vi "Process Job.vi"(8 "error in (no error)":errorcluster, 10 "Task":refnum<class>, 11 "Cashier in":refnum<class "Cashier.lvclass">) -> (0 "error out":errorcluster, 3 "Cashier out":refnum<class "Cashier.lvclass">)   [LabVIEW 2023, in "Cashier.lvclass"]
doc: "Perform the task assigned by the work dispatcher. This VI is an override of a generic method all descendants of the Worker class must implement. \n\nThis method, being implemented by the Cashier class, handles the taking of an order from a Customer."
uses:
  Cashier.lvclass
  Order/Order.lvclass
  Customer Messages/Update order number Msg/Update order number Msg.lvclass/Update order number Msg.ctl
  <vilib>/ActorFramework/Message Enqueuer/Message Enqueuer.lvclass/Message Enqueuer.ctl
  Order/Order.lvclass/Order.ctl
  Customer Messages/Pick up Item Msg/Pick up Item Msg.lvclass
  c:/dev/_r/4/eng/lv-core/lvpostprocessingd/lv_mc_x86_64/dist_i386/vi.lib/ActorFramework/Message/Message.lvclass
  <vilib>/ActorFramework/Self-Addressed Msg/Self-Addressed Msg.lvclass/Self-Addressed Msg.ctl
  Work Dispatcher Messages/Add Task Msg/Add Task Msg.lvclass/Add Task Msg.ctl
  <vilib>/ActorFramework/Message Enqueuer/Enqueue.vi
  Customer Messages/Update order number Msg/Update order number Msg.lvclass
  Work Dispatcher Messages/Add Task Msg/Add Task Msg.lvclass
  <vilib>/ActorFramework/Message Priority Queue/Priority Enqueue.vi
  <vilib>/ActorFramework/Self-Addressed Msg/Self-Addressed Msg.lvclass
  Worker.lvclass
  Order/Order Item.lvclass
panel:
  in  "Ordered Item":string="Ordered item %d/%d..."
  in  "Taking Order":string="Taking order..."
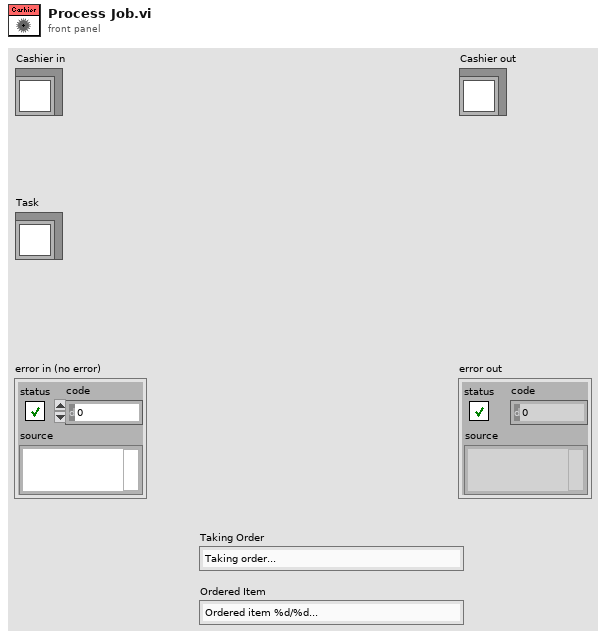
[diagram p1: front panel]
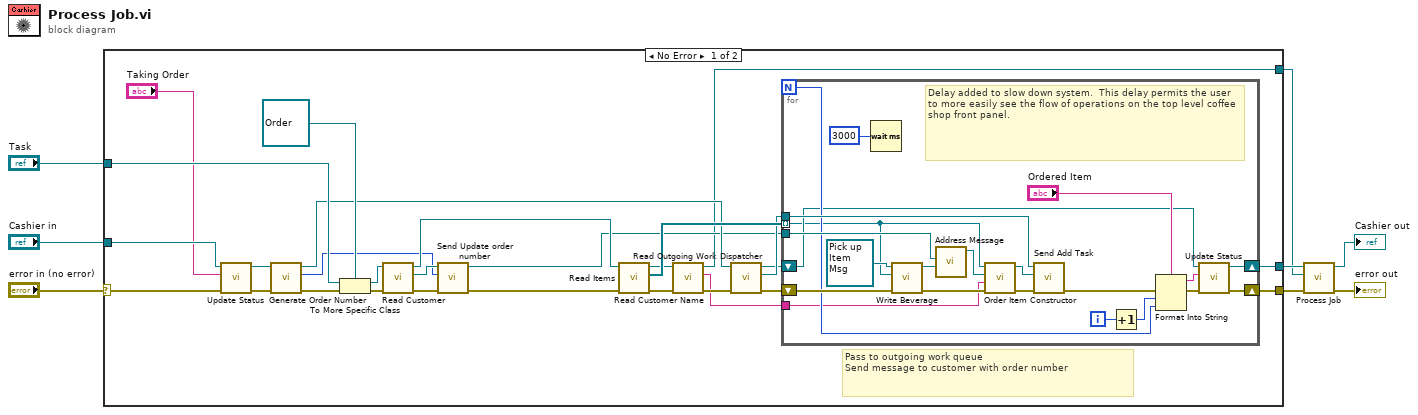
[diagram p0: block diagram]
diagram:
  n1 = case shown="No Error" "error in (no error)" {
    selector: "error in (no error)" -> [w20 w61]
    tunnel: [w25 w61] -> w5
    tunnel: [w14 w60] -> w2
    tunnel: "Cashier in" -> [w18 w60]
    tunnel: "Task" -> [w34 w59]
    tunnel: [w11 w59] -> w1
    frame No Error {
      # "Pass to outgoing work queue\nSend message to customer with order number"
      n2 = call-dynamic "Update Status.vi"("error in (no error)"=w20, "Status"="Taking Order", "Worker in"=w18) -> ("error out"=w19:errorcluster, "Worker out"=w16:refnum<class "Cashier.lvclass">)  [unwired: 7 in]
      n3 = call-dynamic "Generate Order Number.vi"("error in (no error)"=w19, "Cashier in"=w16) -> ("error out"=w24:errorcluster, "Order Number"=w22:u32, "Cashier out"=w23:refnum<class "Cashier.lvclass">)  [unwired: 7 in]
      n4 = To More Specific Class(target class=refnum<class "Order.lvclass"> refnum ("Order in"), reference=w34, error in=w24) -> (specific class reference=w32:refnum<class "Order.lvclass">, error out=w31:errorcluster)
      n5 = call-dynamic "Read Customer.vi"("error in (no error)"=w31, "Order in"=w32) -> ("error out"=w35:errorcluster, "Actor Framework.lvlib:Message Enqueuer"=w36:refnum<class "Message Enqueuer.lvclass">, "Order out"=w29:refnum<class "Order.lvclass">)  [unwired: 7 in]
      n6 = call "Send Update order number.vi"("error in (no error)"=w35, "Order Number"=w22, "Message Enqueuer"=w36) -> ("error out"=w30:errorcluster, "Message Enqueuer out"=w21:refnum<class "Message Enqueuer.lvclass">)  [unwired: 7 in]
      n7 = call-dynamic "Read Items.vi"("error in (no error)"=w30, "Order in"=w29) -> ("error out"=w12:errorcluster, "Items"=w28:refnum<class "Beverage.lvclass">[], "Order out"=w13:refnum<class "Order.lvclass">)  [unwired: 7 in]
      n8 = call "Read Customer Name.vi"("error in (no error)"=w12, "Order in"=w13) -> ("error out"=w10:errorcluster, "Customer Name"=w9:string, "Order out"=w11:refnum<class "Order.lvclass">)  [unwired: 7 in]
      n9 = call-dynamic "Read Outgoing Work Dispatcher.vi"("error in (no error)"=w10, "Worker in"=w23) -> ("error out"=w26:errorcluster, "Actor Framework.lvlib:Message Enqueuer"=w27:refnum<class "Message Enqueuer.lvclass">, "Worker out"=w15:refnum<class "Cashier.lvclass">)  [unwired: 7 in]
      n10 = for {
        N -> [w44]
        tunnel: w28 -> [w39] mode=indexing
        tunnel: w27 -> [w58]
        shift-right: [w42] -> w25
        shift-left: w26 -> [w55]
        tunnel: w21 -> [w53]
        shift-right: [w41] -> w14
        shift-left: w15 -> [w40]
        tunnel: w9 -> [w37]
        i -> [w46]
        # "Delay added to slow down system.  This delay permits the user to more easily see the flow of operations on the top level coffee shop front panel."
        n11 = Wait (ms)(milliseconds to wait=u32 3000) -> ()  [unwired: 1 out]
        n12 = call-dynamic "Write Beverage.vi"("error in (no error)"=w55, "Beverage.lvlib:Beverage.lvclass"=w39, "Pick up Item Msg in"=refnum<class "Pick up Item Msg.lvclass"> refnum) -> ("error out"=w54:errorcluster, "Pick up Item Msg out"=w51:refnum<class "Pick up Item Msg.lvclass">)  [unwired: 7 in]
        n13 = call <vilib>:"Address Message.vi"("Message"=w51, "Destination"=w53) -> ("Self-Addressed Message"=w38:refnum<class "Self-Addressed Msg.lvclass">)  [unwired: 9 in]
        n14 = call "Order Item Constructor.vi"("error in (no error)"=w54, "Cust Name"=w37, "Callback Message"=w38, "Beverage"=w39) -> ("error out"=w57:errorcluster, "Order Item"=w56:refnum<class "Order Item.lvclass">)  [unwired: 6 in]
        n15 = call "Send Add Task.vi"("error in (no error)"=w57, "Task"=w56, "Message Enqueuer"=w58) -> ("error out"=w43:errorcluster)  [unwired: 7 in, 1 out]
        n16 = Increment(x=w46) -> (x+1=w45:i32)
        n17 = Format Into String(format string="Ordered Item", error in=w43, w45, w44) -> (resulting string=w48:string, error out=w49:errorcluster)  [unwired: 1 in]
        n18 = call-dynamic "Update Status.vi"("error in (no error)"=w49, "Status"=w48, "Worker in"=w40) -> ("error out"=w42:errorcluster, "Worker out"=w41:refnum<class "Cashier.lvclass">)  [unwired: 7 in]
      }
    }
    frame Error {
    }
  }
  n19 = call-parent "Process Job.vi"("error in"=w5, "Task"=w1, "Worker in"=w2) -> ("error out"=→"error out":errorcluster, "Worker out"=→"Cashier out":refnum<class "Cashier.lvclass">)  [unwired: 7 in]
